vi "lesson1.vi"() -> ()   [LabVIEW 2020]
panel:
  out "Numeric":dbl
  in  "B":dbl
  in  "A":dbl
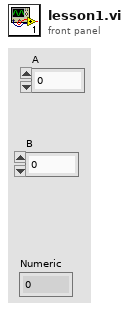
[diagram p1: front panel]
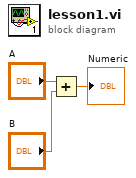
[diagram p0: block diagram]
diagram:
  n1 = Add(x="A", y="B") -> (x+y=→"Numeric":dbl)
